vi "Connection.vi"(6 "Parameters":variant, 7 "Timeout":i32=5000, 8 "error in (no error)":errorcluster, 9 "Port":u16=102, 10 "IP Address":string, 11 "SIMATIC_S7 in":refnum<class "SIMATIC_S7.lvclass">) -> (0 "error out":errorcluster, 3 "SIMATIC_S7 out":refnum<class "SIMATIC_S7.lvclass">)   [LabVIEW 2025, in "SIMATIC_S7.lvclass"]
uses:
  SIMATIC_S7.lvclass
  <vilib>/Hampel Software Engineering/S7NetCom/Source/Controls/PDU Size--ring.ctl
  SIMATIC_S7.lvclass/SIMATIC_S7.ctl
  <vilib>/Hampel Software Engineering/S7NetCom/Source/S7NetCom.lvclass
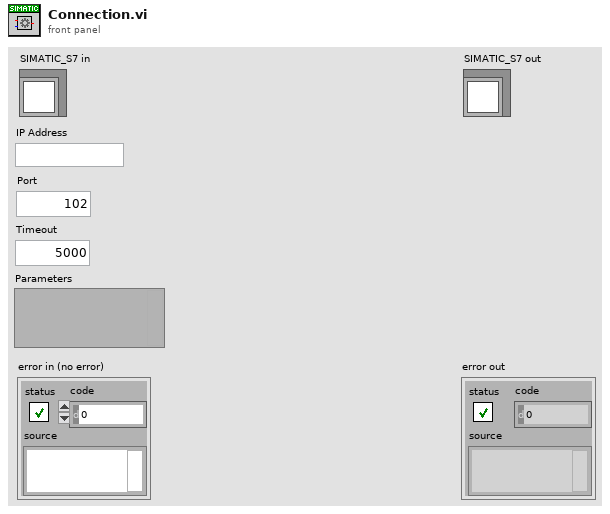
[diagram p1: front panel]
types:
  T1 = typedef "S7NetCom.lvlib/S7NetCom.lvclass/PDU Size--ring.ctl" = u16
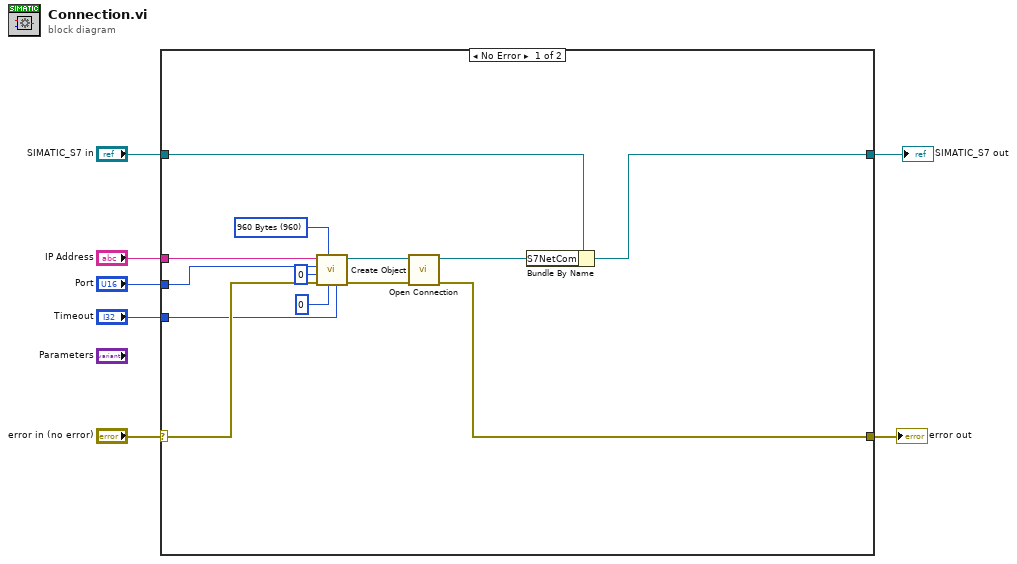
[diagram p0: block diagram]
diagram:
  n1 = case shown="No Error" "error in (no error)" {
    selector: "error in (no error)" -> [w17 w21]
    tunnel: "SIMATIC_S7 in" -> [w18 w22]
    tunnel: [w14 w22] -> w5
    tunnel: [w16 w21] -> w4
    tunnel: "IP Address" -> [w13 _]
    tunnel: "Port" -> [w12 _]
    tunnel: "Timeout" -> [w11 _]
    frame No Error {
      w9 = T1 960 items=["240 Bytes"=240, "480 Bytes"=480, "960 Bytes"=960] ("PDU Size")
      n2 = call <vilib>:"Create Object.vi"("Timeout"=w11, "Rack"=u8 0, "PDU Size"=w9, "error in"=w17, "Slot"=u8 0, "Port"=w12, "IP Address"=w13) -> ("error out"=w19:errorcluster, "S7NetCom out"=w20:refnum<class "S7NetCom.lvclass">)  [unwired: 3 in]
      n3 = call <vilib>:"Open Connection.vi"("error in"=w19, "S7NetCom in"=w20) -> ("error out"=w16:errorcluster, "S7NetCom out"=w15:refnum<class "S7NetCom.lvclass">)  [unwired: 8 in]
      n4 = Bundle By Name(cluster=w18, "S7NetCom"=w15) -> (w14:refnum<class "SIMATIC_S7.lvclass">)
    }
    frame Error {
    }
  }
  "error out" <- w4
  "SIMATIC_S7 out" <- w5
